vi "STB.vi"(8 "error in (no error)":errorcluster, 10 "Node In":string, 11 "VISA resource name":refnum<visa-resource-name>) -> (0 "error out":errorcluster, 1 "STB":u8, 2 "Node Out":string, 3 "VISA resource name out":refnum<visa-resource-name>, 4 "Command String":string)   [LabVIEW 2009, in "Keithley 2600 Series.lvlib"]
doc: "Status Byte Register query. *STB?\n\n<b>Functions and Attributes Used</b>\nstatus.condition"
uses:
  <instrlib>/Keithley 2600 Series/Keithley 2600 Series.lvlib
panel:
  # "(c) 2008 Keithley Instruments, Inc.  ALL RIGHTS RESERVED."
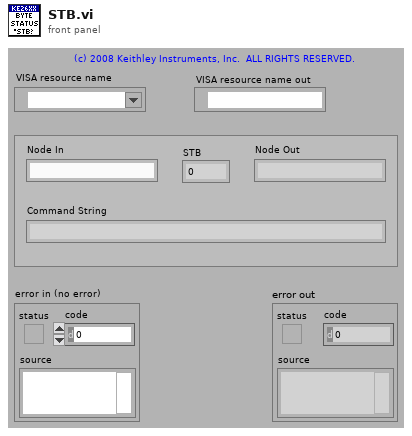
[diagram p1: front panel]
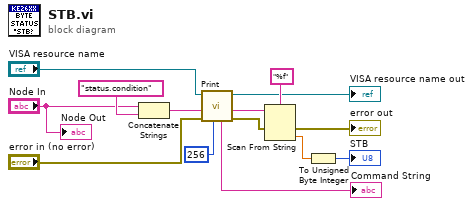
[diagram p0: block diagram]
diagram:
  n1 = Concatenate Strings("Node In", "status.condition" ("string")) -> (w12:string)
  n2 = call <instrlib>:"Print.vi"("Byte Count (1024)"=u32 256, "error in (no error)"="error in (no error)", "Input"=w12, "VISA resource name"="VISA resource name") -> ("error out"=w7:errorcluster, "Output"=w9:string, "VISA resource name out"=→"VISA resource name out":refnum<visa-resource-name>, "Command String"=→"Command String":string)  [unwired: 1 in, 3 out]
  n3 = Scan From String(format string="%f", input string=w9, error in=w7) -> (error out=→"error out":errorcluster, output 1=w6:dbl)  [unwired: 1 in, 3 out]
  n4 = To Unsigned Byte Integer(number=w6) -> (unsigned 8bit integer=→"STB":u8)
  "Node Out" <- "Node In"
